vi "I2C Init.vi"(4 "SDA GPIO":T2=-1, 6 "SCL GPIO":T2=-1, 7 "I2C #":T1=-1, 8 "error in (no error)":errorcluster, 10 "Baud":u32=400000 format="%.0p", 11 "VisaComms in":refnum<class "VisaComms.lvclass">) -> (0 "error out":errorcluster, 3 "VisaComms out":refnum<class "VisaComms.lvclass">)   [LabVIEW 2020, in "CTI.lvlib" / "VisaComms.lvclass"]
uses:
  VisaComms.lvclass
  GPIO Number.ctl
  I2C Number.ctl
  VisaComms.lvclass/VisaComms.ctl
  CTI.lvlib
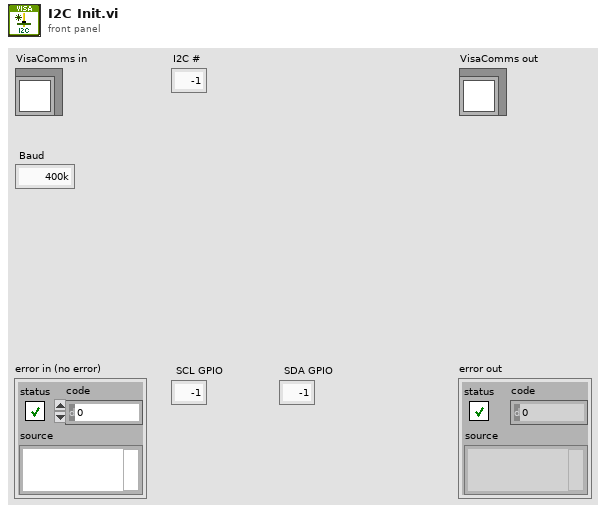
[diagram p1: front panel]
types:
  T1 = typedef "CTI.lvlib/I2C Number.ctl" = i8
  T2 = typedef "CTI.lvlib/GPIO Number.ctl" = i8
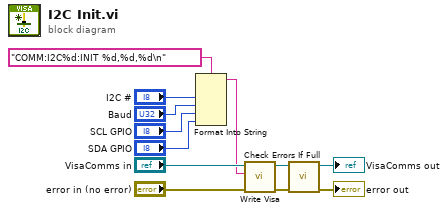
[diagram p0: block diagram]
diagram:
  n1 = Format Into String(format string="COMM:I2C%d:INIT %d,%d,%d\n", "I2C #", "Baud", "SCL GPIO", "SDA GPIO") -> (resulting string=w5:string)  [unwired: 2 in, 1 out]
  n2 = call "Write Visa.vi"("error in (no error)"="error in (no error)", "write buffer"=w5, "VisaComms in"="VisaComms in") -> ("error out"=w4:errorcluster, "VisaComms out"=w2:refnum<class "VisaComms.lvclass">)  [unwired: 6 in, 1 out]
  n3 = call "Check Errors If Full.vi"("error in (no error)"=w4, "VisaComms in"=w2) -> ("error out"=→"error out":errorcluster, "VisaComms out"=→"VisaComms out":refnum<class "VisaComms.lvclass">)  [unwired: 8 in]
